vi "state graph.vi"(3 "Clear graph":bool, 4 "sensor to plot":i32=3, 5 "Plant Method":T1={"Operator information"=[], "data log interval"=60, "data loop interval"=10, "Datalog directory path"=path "", "graph update interval"=1.0, "history length"=1000, "Control Logic file path"=path "", "Sensor Configuration file path"=path "", "HMI VI path"=path "", "HMI data smooth"=5.0} {"HMI data smooth" min=0.01 format="%.2f"; "history length" min=1; "graph update interval" min=0.1 format="%.2f"; "data log interval" min=1}) -> (0 "Sensor Data Smoothed":T3 {"Sensor array"."scaled" format="%.2f"; "Sensor array"."voltage" format="%.4f"; "Time" format="%<%I:%M:%S%2u %p\n%m/%d/%Y>T"}, 1 "state graph":cluster{dbl[], dbl[]}, 2 "sensor graph":cluster{dbl[], dbl[]})   [LabVIEW 2012]
uses:
  TCP DAQ/Sensor data.ctl
  DAQ configuration/sensor cluster.ctl
  Plant method.ctl
  operator info.ctl
  DAQ configuration/Sensor buffer command.ctl
  logic buffer cmd.ctl
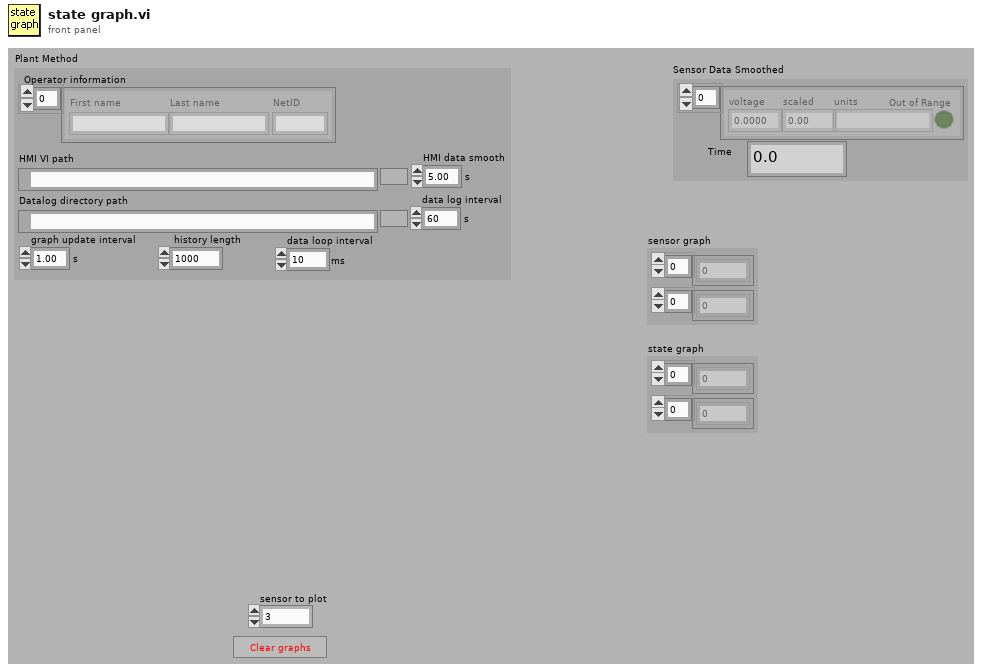
[diagram p1: front panel]
types:
  T1 = typedef "Plant method.ctl" = cluster{"Operator information":T2, "data log interval":u32, "data loop interval":u32, "Datalog directory path":path, "graph update interval":sgl, "history length":u16, "Control Logic file path":path, "Sensor Configuration file path":path, "HMI VI path":path, "HMI data smooth":dbl}
  T2 = typedef "operator info.ctl" = cluster{"First name":string, "Last name":string, "NetID":string}[]
  T3 = typedef "Sensor data.ctl" = cluster{" Sensor array":T4[], "Time":dbl}
  T4 = typedef "sensor cluster.ctl" = cluster{"voltage":sgl, "scaled":sgl, "units":string, "Out of Range":bool}
  T5 = typedef "logic buffer cmd.ctl" = enum16{"read", "write ouput settings", "write rules", "write setpoints", "write output descriptions", "write all", "calculate setpoints", "save", "open", "Load all setpoint code", "Load one setpoint code", "Configure one setpoint code"}
  T6 = typedef "Sensor buffer command.ctl" = enum16{"read average", "read recent", "read all", "write", "configure", "clear"}
  T7 = typedef "variable setpoint.ctl" = cluster{"name":string, "unit":string, "value":dbl, "Type":enum16{"Constant", "Variable"}, "variable":cluster{"selected sensors":i32[], "selected set points":i32[], "VI":path, "Data average interval":T8, "code ref":T9}}
  T8 = typedef "data ave interval.ctl" = dbl
  T9 = typedef "type specifier for control code.ctl" = refnum<vi>
  T10 = typedef "Plant state.ctl" = u16
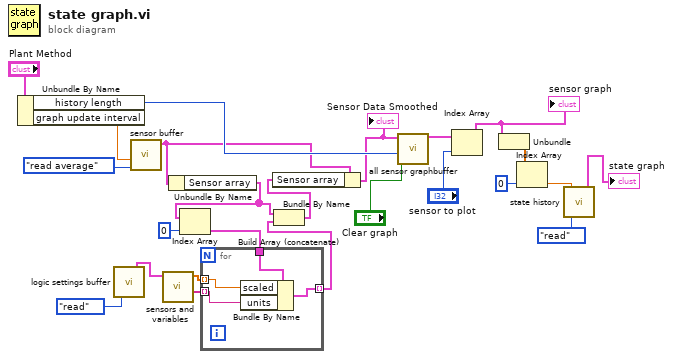
[diagram p0: block diagram]
diagram:
  n1 = Unbundle By Name("Plant Method") -> ("history length"=w6:u16, "graph update interval"=w20:sgl)
  n2 = call "logic settings buffer.vi"("command"=logic_buffer_cmd."read") -> ("Set Points out"=w11:T7[])  [unwired: 11 in, 7 out]
  n3 = call "sensor buffer.vi"("command"=Sensor_buffer_command."read average", "smooth interval (s)"=w20) -> ("Sensor Data smoothed"=w5:T3)  [unwired: 3 in, 2 out]
  n4 = call "sensors and variables.vi"("S P & V definitions"=w11) -> ("units"=w7:string[], "Variable values"=w8:dbl[])  [unwired: 7 in, 2 out]
  n5 = Unbundle By Name(w5) -> ("Sensor array"=w4:T4[])
  n6 = Index Array(array=w4, index=0) -> (element=w9:T4)
  n7 = for {
    tunnel: w9 -> [w28]
    tunnel: w8 -> [w27] mode=indexing
    tunnel: w7 -> [w26] mode=indexing
    tunnel: [w25] -> w3 mode=indexing
    n8 = Bundle By Name(cluster=w28, "scaled"=w27, "units"=w26) -> (w25:T4)
  }
  n9 = Build Array (concatenate)(w4, w3) -> (w2:T4[])
  n10 = Bundle By Name(cluster=w5, "Sensor array"=w2) -> (w1:T3)
  "Sensor Data Smoothed" <- w1
  n11 = call "all sensor graphbuffer.vi"("Reset"="Clear graph", "history length"=w6, "Sensor Data"=w1) -> ("Multiplot graph data"=w23:cluster{dbl[], dbl[]}[])  [unwired: 6 in, 2 out]
  n12 = Index Array(array=w23, index="sensor to plot") -> (element=w15:cluster{dbl[], dbl[]})
  "sensor graph" <- w15
  n13 = Unbundle(w15) -> (w18:dbl[])  [unwired: 1 out]
  n14 = Index Array(array=w18, index=0) -> (element=w16:dbl)
  n15 = call "state history.vi"("command"=enum16{"write", "read", "reset"}."read", "Time"=w16) -> ("state history"=→"state graph":cluster{dbl[], T10[]})  [unwired: 1 in]
